vi "Pulse Mode - Set Configurations.vi"   [LabVIEW 2014, in "Associated Power Technologies 8500 Series.lvlib"]
uses:
  <instrlib>/Associated Power Technologies 8500 Series/Associated Power Technologies 8500 Series.lvlib
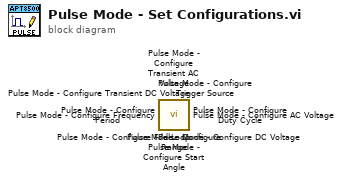
[diagram p0: block diagram]
diagram:
  n1 = call <instrlib>:"Pulse Mode - Configure Range.vi"() -> ()  [unwired: 10 in, 2 out]
  n2 = call <instrlib>:"Pulse Mode - Configure Trigger Source.vi"() -> ()  [unwired: 10 in, 2 out]
  n3 = call <instrlib>:"Pulse Mode - Configure Period.vi"() -> ()  [unwired: 10 in, 2 out]
  n4 = call <instrlib>:"Pulse Mode - Configure Duty Cycle.vi"() -> ()  [unwired: 10 in, 2 out]
  n5 = call <instrlib>:"Pulse Mode - Configure Transient DC Voltage.vi"() -> ()  [unwired: 10 in, 2 out]
  n6 = call <instrlib>:"Pulse Mode - Configure Transient AC Voltage.vi"() -> ()  [unwired: 10 in, 2 out]
  n7 = call <instrlib>:"Pulse Mode - Configure Start Angle.vi"() -> ()  [unwired: 10 in, 2 out]
  n8 = call <instrlib>:"Pulse Mode - Configure DC Voltage.vi"() -> ()  [unwired: 10 in, 2 out]
  n9 = call <instrlib>:"Pulse Mode - Configure Frequency.vi"() -> ()  [unwired: 10 in, 2 out]
  n10 = call <instrlib>:"Pulse Mode - Configure AC Voltage.vi"() -> ()  [unwired: 10 in, 2 out]
  n11 = call <instrlib>:"Pulse Mode - Configure File Loop.vi"() -> ()  [unwired: 10 in, 2 out]
